vi "Get PanelBouds.vi"(8 "error in (no error)":errorcluster caption="错误输入（无错误）", 11 "PanelDataNode 输入":refnum<class "PanelDataNode.lvclass"> caption="DNL_LabVIEW Object in") -> (0 "error out":errorcluster caption="错误输出", 2 "Bounds":T1, 3 "PanelDataNode 输出":refnum<class "PanelDataNode.lvclass"> caption="DNL_LabVIEW Object out")   [LabVIEW 2013, in "PanelDataNode.lvclass"]
uses:
  PanelDataNode.lvclass
  <vilib>/Utility/miscctls.llb/LVBoundsTypeDef.ctl
  PanelDataNode.lvclass/PanelDataNode.ctl
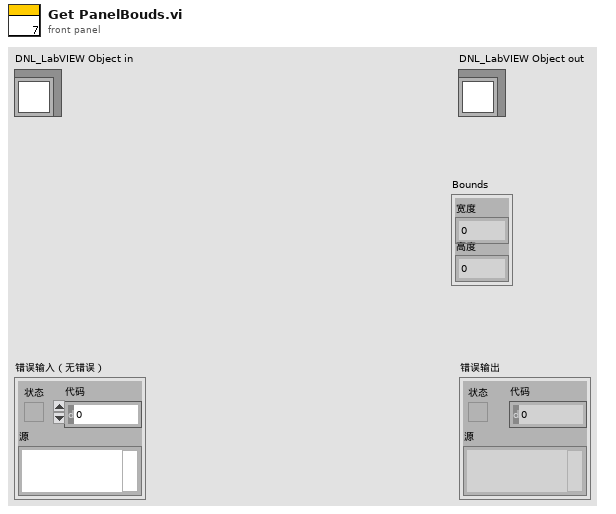
[diagram p1: front panel]
types:
  T1 = typedef "LVBoundsTypeDef.ctl" = cluster{"Width":u32, "Height":u32}
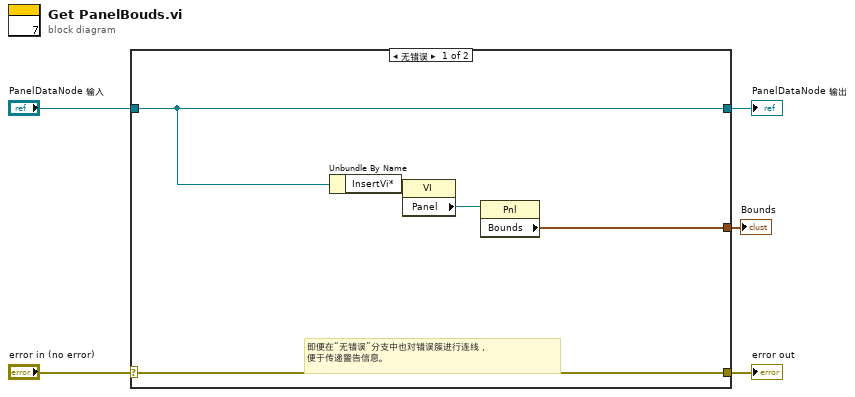
[diagram p0: block diagram]
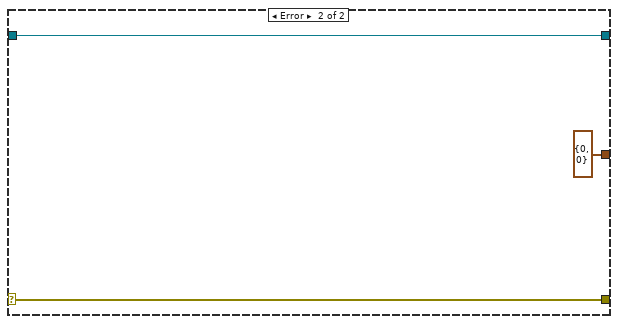
[diagram p2: hidden frame]
diagram:
  n1 = case shown="无错误" "error in (no error)" {
    selector: "error in (no error)" -> [w10 w13]
    tunnel: [w10 w13] -> w4
    tunnel: [w9 w12] -> w2
    tunnel: "PanelDataNode 输入" -> [w9 w12]
    tunnel: [w6 T1 {"Width"=0, "Height"=0} ("Bounds")] -> w1
    frame No Error {
      # "即便在“无错误”分支中也对错误簇进行连线，\n便于传递警告信息。"
      n2 = Unbundle By Name(w9) -> ("InsertVi*"=w8:refnum<vi>)
      n3 = property class="VI"(reference=w8) -> ("Panel"=w7:refnum<vi>)  [unwired: 1 in, 2 out]
      n4 = property class="Pnl"(reference=w7) -> ("Bounds"=w6:T1)  [unwired: 1 in, 2 out]
    }
    frame Error {
    }
  }
  "error out" <- w4
  "PanelDataNode 输出" <- w2
  "Bounds" <- w1
